vi "Get Pot Value.vi"(10 "Side":enum16{"Left", "Right"}(ring), 11 "arm.lvclass":refnum<class "arm.lvclass">) -> (2 "Value":dbl, 3 "arm.lvclass":refnum<class "arm.lvclass">)   [LabVIEW 2015, in "arm.lvclass"]
uses:
  arm.lvclass
  arm.lvclass/arm.ctl
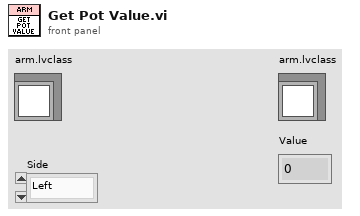
[diagram p1: front panel]
types:
  T1 = typedef "WPI_PotentiometerDevRef.ctl" = cluster{"DevStatus":errorcluster, "Analog Channel":T2, "Invert Output":bool}
  T2 = typedef "FPGA_AIChannel.ctl" = enum8{"AI 0", "AI 1", "AI 2", "AI 3", "AI MXP 0", "AI MXP 1", "AI MXP 2", "AI MXP 3", "Invalid"}
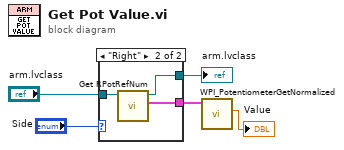
[diagram p0: block diagram]
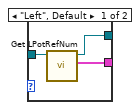
[diagram p2: hidden frame]
diagram:
  n1 = case shown="\"Right\"" "Side" {
    tunnel: "arm.lvclass" -> [w8 w9]
    tunnel: [w7 w10] -> w5
    tunnel: [w6 w11] -> w4
    frame "Left", Default {
      n2 = call "Get LPotRefNum.vi"("arm in"=w8) -> ("PotDevRef"=w7:T1, "arm out"=w6:refnum<class "arm.lvclass">)  [unwired: 9 in]
    }
    frame "Right" {
      n3 = call "Get RPotRefNum.vi"("arm in"=w9) -> ("PotDevRef"=w10:T1, "arm out"=w11:refnum<class "arm.lvclass">)  [unwired: 9 in]
    }
  }
  "arm.lvclass" <- w4
  n4 = call <vilib>:"WPI_PotentiometerGetNormalized.vi"("PotDevRef"=w5) -> ("Normalized Value"=→"Value":dbl)  [unwired: 8 in, 2 out]
